vi "EscapeHTMLCharacters.vi"(10 "String":string) -> (2 "Escaped String":string)   [LabVIEW 2020, in "DP_WebView.lvclass"]
uses:
  DP_WebView.lvclass
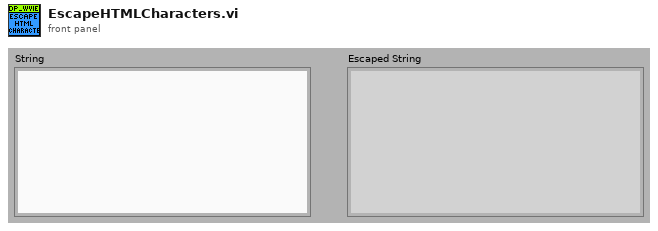
[diagram p1: front panel]
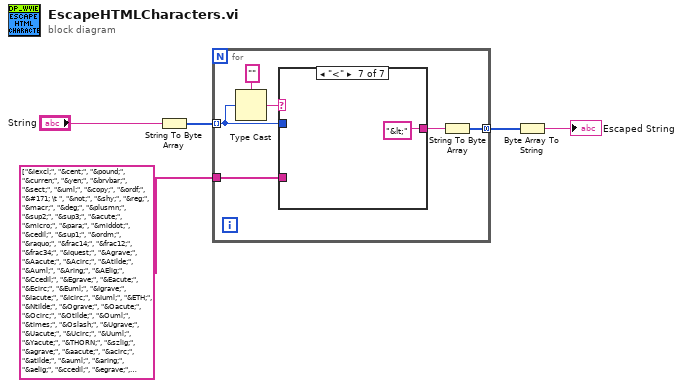
[diagram p0: block diagram]
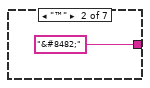
[diagram p3: hidden frame]
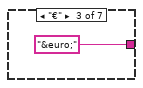
[diagram p4: hidden frame]
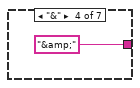
[diagram p5: hidden frame]
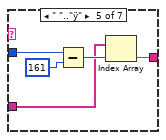
[diagram p6: hidden frame]
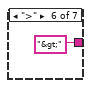
[diagram p7: hidden frame]
diagram:
  n1 = String To Byte Array(string="String") -> (unsigned byte array=w3:u8[])
  n2 = for {
    tunnel: w3 -> [w7] mode=indexing
    tunnel: [w8] -> w2 mode=concatenating
    tunnel: string[] ["&iexcl;", "&cent;", "&pound;", "&curren;", "&yen;", "&brvbar;", "&sect;", "&uml;", "&copy;", "&ordf;", "&#171; \t ", "&not;", "&shy;", "&reg;", "&macr;", "&deg;", "&plusmn;", "&sup2;", "&sup3;", "&acute;", "&micro;", "&para;", "&middot;", "&cedil;", "&sup1;", "&ordm;", "&raquo;", "&frac14;", "&frac12;", "&frac34;", "&iquest;", "&Agrave;", "&Aacute;", "&Acirc;", "&Atilde;", "&Auml;", "&Aring;", "&AElig;", "&Ccedil;", "&Egrave;", "&Eacute;", "&Ecirc;", "&Euml;", "&Igrave;", "&Iacute;", "&Icirc;", "&Iuml;", "&ETH;", "&Ntilde;", "&Ograve;", "&Oacute;", "&Ocirc;", "&Otilde;", "&Ouml;", "&times;", "&Oslash;", "&Ugrave;", "&Uacute;", "&Ucirc;", "&Uuml;", "&Yacute;", "&THORN;", "&szlig;", "&agrave;", "&aacute;", "&acirc;", "&atilde;", "&auml;", "&aring;", "&aelig;", "&ccedil;", "&egrave;", "&eacute;", "&ecirc;", "&euml;", "&igrave;", "&iacute;", "&icirc;", "&iuml;", "&eth;", "&ntilde;", "&ograve;", "&oacute;", "&ocirc;", "&otilde;", "&ouml;", "&divide;", "&oslash;", "&ugrave;", "&uacute;", "&ucirc;", "&uuml;", "&yacute;", "&thorn;"] ("Array of Strings") -> [w6]
    n3 = Type Cast(type="", x=w7) -> (*(type *) &x=w10:string)
    n4 = case shown="\"<\"" w10 {
      selector: w10 -> [w12 _ _ _ _ _ _]
      tunnel: [w12 "&#8482;" "&euro;" "&amp;" w16 "&gt;" ("search string") "&lt;" ("search string")] -> w9
      tunnel: w7 -> [_ _ _ _ w20 _ _]
      tunnel: w6 -> [_ _ _ _ w17 _ _]
      frame Default {
      }
      frame "™" {
      }
      frame "€" {
      }
      frame "&" {
      }
      frame " ".."ÿ" {
        n5 = Subtract(x=w20, y=u8 161) -> (x-y=w18:u8)
        n6 = Index Array(array=w17, index=w18) -> (element=w16:string)
      }
      frame ">" {
      }
      frame "<" {
      }
    }
    n7 = String To Byte Array(string=w9) -> (unsigned byte array=w8:u8[])
  }
  n8 = Byte Array To String(unsigned byte array=w2) -> (string=→"Escaped String":string)
